vi "test Get and Set TX Duration.vi"(8 "error in (no error)":errorcluster, 11 "TestCase in":refnum<class "Framework Status Tests.lvclass">) -> (0 "error out":errorcluster, 3 "TestCase out":refnum<class "Framework Status Tests.lvclass">)   [LabVIEW 2017, in "Framework Status Tests.lvclass"]
uses:
  Framework Status Tests.lvclass
  Engine/Classes/Status/Framework Performance.lvclass/Framework Performance.ctl
  <vilib>/NI/Memory Manager/Classes/Pointer/Pointer.lvclass/Pointer.ctl
  <vilib>/NI/Memory Manager/Classes/Pointer/API/Write Pointer Data.vi
  <vilib>/NI/Memory Manager/Classes/Pointer/Public/Write/Write (0D U32).vi
  <vilib>/NI/Memory Manager/Classes/Pointer/API/Read Pointer Data.vi
  <vilib>/NI/Memory Manager/Classes/Pointer/Public/Read/Read (0D U32).vi
  <vilib>/NI/Memory Manager/Classes/Pointer/Public/Write (No Check)/Write (No Check 0D U32).vi
  <vilib>/NI/Memory Manager/Classes/Pointer/Protected/Parameter Checking/Check Null Pointer.vi
  <vilib>/NI/Memory Manager/Classes/Pointer/Protected/Parameter Checking/Check Subset.vi
  <vilib>/NI/Memory Manager/Classes/Pointer/Public/Read (No Check)/Read (No Check 0D U32).vi
  <vilib>/NI/Memory Manager/Classes/Pointer/API/Accessors/Get Address.vi
  <vilib>/NI/Memory Manager/Classes/Pointer/Protected/Errors.vi
  <vilib>/NI/Memory Manager/Classes/Pointer/Protected/Error VIs/Null Pointer.vi
  <vilib>/NI/Memory Manager/Classes/Pointer/Protected/Error VIs/Out of Bounds.vi
  <vilib>/NI/Memory Manager/Classes/Pointer/API/Accessors/Get Size.vi
  <vilib>/NI/Memory Manager/Classes/Pointer/Protected/Error Building/Create Error.vi
  <vilib>/NI/Memory Manager/VIs/Write String into Source.vi
  <vilib>/NI/Memory Manager/Classes/Pointer/Protected/Error Building/Write Pointer Size.vi
  <vilib>/NI/Memory Manager/VIs/Write Number into Source.vi
  <vilib>/NI/Memory Manager/VIs/VIs for Poly/Write U64 into Source.vi
  <vilib>/NI/Memory Manager/Constants/Constants.vi
  <vilib>/NI/Memory Manager/Constants/Library Name.vi
  <vilib>/NI/Memory Manager/Classes/Pointer/Protected/Error Building/Get Error Info.vi
  <vilib>/NI/Memory Manager/VIs/Create Error Cluster.vi
  <vilib>/NI/Memory Manager/VIs/VIs for Poly/Create Error Cluster (256B).vi
  <vilib>/NI/Memory Manager/VIs/Set Error Status.vi
  <vilib>/NI/Memory Manager/VIs/Set Error Code.vi
  <vilib>/NI/Memory Manager/VIs/Set Error Source.vi
  <vilib>/addons/_JKI Toolkits/VI Tester/TestCase.llb/TestCase.lvclass
  Engine/Classes/Status/Framework Performance.lvclass
  C:/Program Files (x86)/National Instruments/LabVIEW 2017/vi.lib/addons/_JKI Toolkits/VI Tester/TestCase.llb/TestCase.lvclass
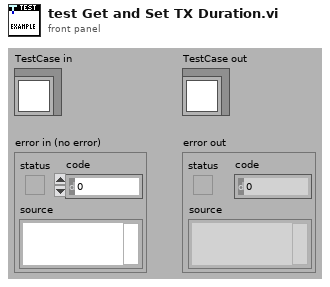
[diagram p1: front panel]
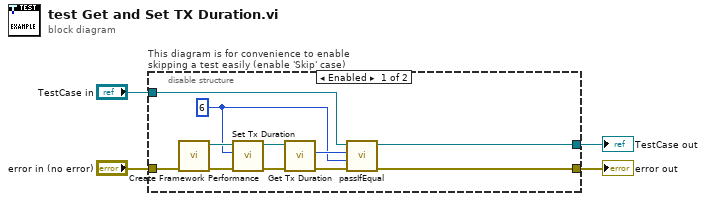
[diagram p0: block diagram]
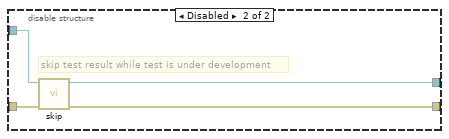
[diagram p2: hidden frame]
diagram:
  n1 = disable-structure "This diagram is for convenience to enable skipping a test easily (enable 'Skip' case)" shown="Enabled" {
    disable-tunnel: "TestCase in" -> [w14 w19]
    disable-tunnel: [w13 w17] -> w1
    disable-tunnel: [w15 w18] -> w3
    disable-tunnel: "error in (no error)" -> [w6 w16]
    frame Enabled {
      w7 = u32 6 ("rx duration")
      n2 = call "Create Framework Performance.vi"("error in (no error)"=w6) -> ("error out"=w10:errorcluster, "Framework Performance"=w12:refnum<class "Framework Performance.lvclass">)  [unwired: 9 in]
      n3 = call "Set Tx Duration.vi"("error in (no error)"=w10, "tx duration"=w7, "Framework Performance in"=w12) -> ("error out"=w9:errorcluster, "Framework Performance out"=w11:refnum<class "Framework Performance.lvclass">)  [unwired: 7 in]
      n4 = call "Get Tx Duration.vi"("error in (no error)"=w9, "Framework Performance in"=w11) -> ("error out"=w5:errorcluster, "tx duration"=w8:u32)  [unwired: 7 in, 1 out]
      n5 = call-dynamic "passIfEqual.vi"("error in (no error)"=w5, "y"=w7, "x"=w8, "TestCase in"=w14) -> ("error out"=w15:errorcluster, "TestCase out"=w13:refnum<class "Framework Status Tests.lvclass">)  [unwired: 6 in]
    }
    frame Disabled {
      # "skip test result while test is under development"
      n6 = call <vilib>:"skip.vi"("error in (no error)"=w16, "TestCase in"=w19) -> ("error out"=w18:errorcluster, "TestCase out"=w17:refnum<class "Framework Status Tests.lvclass">)  [unwired: 8 in]
    }
  }
  "error out" <- w3
  "TestCase out" <- w1
